vi "Return_Last_Result_To_Webservice.vi"(8 "error in (no error)":errorcluster, 10 "String":string, 11 "waveform in":waveform(sgl)) -> (0 "error out":errorcluster, 3 "JSON string":string)   [LabVIEW 2015]
uses:
  Share Data/uPower_kit.ctl
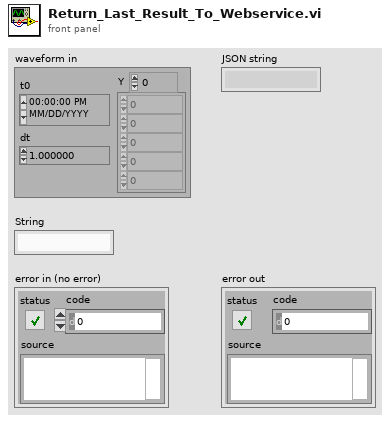
[diagram p1: front panel]
types:
  T1 = typedef "uPower_kit.ctl" = cluster{"DEV":string, "BUSY":bool, "VBAT":dbl, "OUTPUT":bool, "LAST_RESULT":dbl, "DURATION":u16, "TRIGGER":bool, "RANGE":string, "Vsource":dbl, "FW":string, "Mode":string}
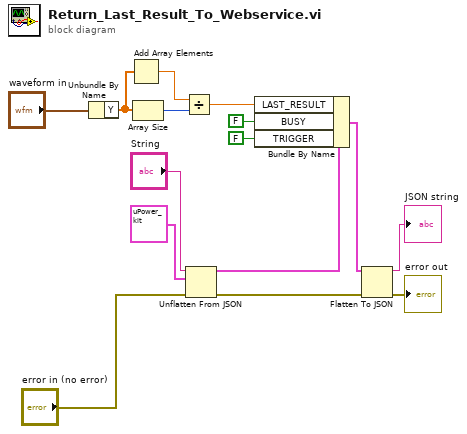
[diagram p0: block diagram]
diagram:
  n1 = Unbundle By Name("waveform in") -> ("Y"=w5:sgl[])
  n2 = Add Array Elements(numeric array=w5) -> (sum=w3:sgl)
  n3 = Array Size(array=w5) -> (size(s)=w2:i32)
  n4 = Divide(x=w3, y=w2) -> (x/y=w8:sgl)
  n5 = Unflatten From JSON(JSON string="String", type and defaults=T1 {"DEV"="", "BUSY"=FALSE, "VBAT"=0.0, "OUTPUT"=FALSE, "LAST_RESULT"=0.0, "DURATION"=0, "TRIGGER"=FALSE, "RANGE"="", "Vsource"=0.0, "FW"="", "Mode"=""} ("DEV_BUSY"), error in (no error)="error in (no error)") -> (value=w1:T1, error out=w14:errorcluster)  [unwired: 4 in]
  n6 = Bundle By Name(cluster=w1, "LAST_RESULT"=w8, "BUSY"=FALSE, "TRIGGER"=FALSE) -> (w11:T1)
  n7 = Flatten To JSON(anything=w11, error in (no error)=w14) -> (JSON string=→"JSON string":string, 11:→"error out":errorcluster)  [unwired: 1 in]
